vi "rqcAlice Key Distribution (Low Level Example).vi"() -> ()   [LabVIEW 2018]
uses:
  Custom Controls/rqcAlice States.ctl
  FPGA/Alice/Custom Controls/Phase Modulator/rqcAlice Mod.Config.ctl
  Shared/Shared FPGA Lib/Shared Logic/Custom Controls/rqc Random Generator.parameters.ctl
  Shared/Shared FPGA Lib/Shared Logic/Custom Controls/rqc Random Generator.value type.ctl
  FPGA/Alice/Custom Controls/Main State Machine/rqcAlice DAC Clock Positions.ctl
  Shared/Shared Host Lib/rqc ServiceNET/Custom Controls/rqc ServiceNET command.ctl
  Shared/Shared Host Lib/rqc ServiceNET/Alice/Custom Controls/rqcAlice ServiceNET control.ctl
  <vilib>/FPGAPlugInAG/PCIe-7820R/niLvFpga_Open_PCIe-7820R.vi
  <vilib>/rvi/interface/common/dynamic/niFpgaDynamicAddResources.vi
  <vilib>/FPGAPlugInAG/Dynamic/niLvFpga_Close_Dynamic.vi
  <vilib>/rvi/interface/nirviOpenFPGA/nirviOpenFPGA.xnode
  FPGA Bitfiles/rqcAlice FPGA (7820R) v 3.2.0.lvbitx
  <vilib>/rvi/interface/nirviCloseFPGA/nirviCloseFPGA.xnode
panel:
  in  "Sessions to Key File":u32
  in  "Write to File QBER threshold":dbl=5.0 format="%#_g %"
  in  "Attenuation, dB":dbl max=40.0
  out "IP Address":string="192.168.0.209"
  in  "DL SD":u32=24674
  in  "Coax/SD":bool
  out "QBER Graph":dbl[](graph)
  in  "pm.off":u8=2
  in  "pm.on":u8=9
  in  "PM\nRandom\nOn/Off":bool=TRUE
  in  "Pi Voltage":u16=160
  out "Real pulse count:":i32=1000000
  out "Total pulses expected:":u32=1000000
  out "QBER, %":dbl=1.8333333333333333
  out "Bob's Key:":string="000001111000001000111001111011010101010110101010000001111011010111010100010111101101000100111011011011100011101010101111010000010101011111010011110111101011110110111011001100100110010000110101011100111010010011100011011100000100000100011001010111010011011011011111001000001100001100101000101111000011101010000011011101000010000001100110010111011010110010111010010100010111010010111010010010101000110110111000000101101000010001111111011110101110001110011010101111011010011001011111000111111101001100010111110011011101111001111000111010111111101001001100001111010010001111001011101101001000000101001010"
  out "Alice's Key:":string="000001111000001000111000111011010101010110101010000001111011010111010100010111101001000110111011011011100011101010101111010010010101011111010011110111101011111110111011001100100110010000110101011100111010010011100011011100000100000100011001110111010011011011011101001000001100001100101000101111000011100010000011011101000010000001100010110111011010110010111010010100010111010010111010010010101000110110111000000101101000010001111111011110101110001110011010101111011010011001011111000111111101001100010111110011011101111001111000111010111111101001001100001111010010001111001011111101001000000101001010"
  in  "Pulses in Train":u32=1000
  in  "Train Number":i32=1000
  in  "DL Coax":u32=24704
  out "error out":errorcluster
  in  "Stop":bool
  out "connected?":bool
  in  "Port":u16=5020
  out "Current State":T1=enum."App.Stop"
  # "ALICE"
  # "LAN settings:"
  # "Data exchange details:"
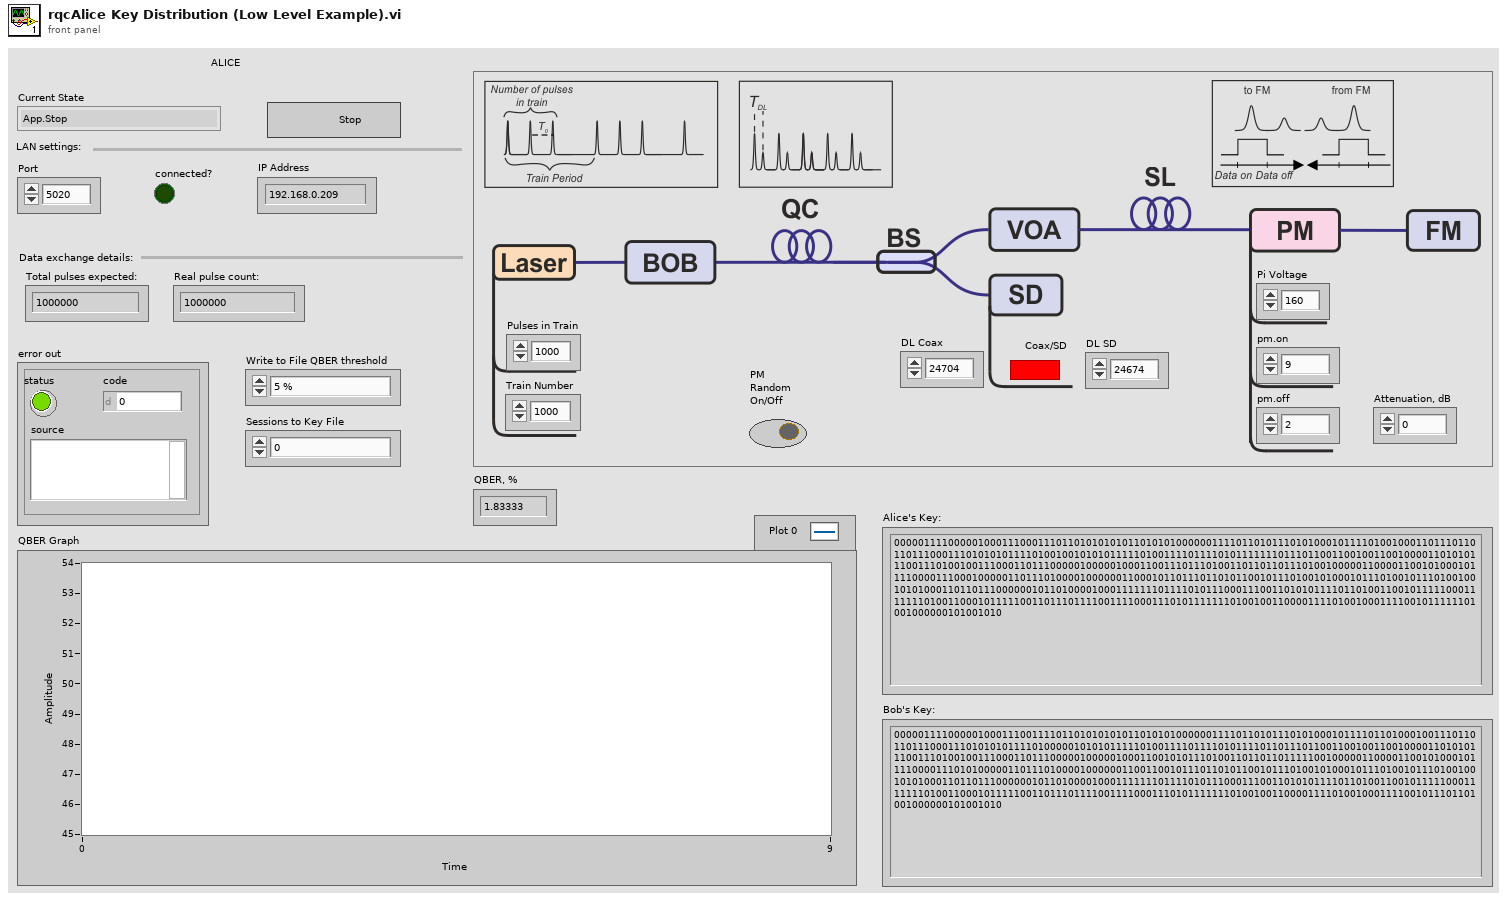
[diagram p1: front panel]
types:
  T1 = typedef "rqcAlice States.ctl" = enum16{"HW.configure", "HW.meas", "NET.create", "NET.connect", "NET.readCommand", "NET.sendCommand", "NET.readData", "NET.close", "Meas.Start", "Meas.NextStep", "Meas.restart", "Meas.Done", "App.HandleEvent", "App.HandleError", "App.Stop"}
  T2 = typedef "rqcAlice DAC Clock Positions.ctl" = u8[]
  T3 = typedef "rqc Random Generator.parameters.ctl" = cluster{"value type":T4, "constant":u16, "num of levels":u16, "levels values":u16[]}
  T4 = typedef "rqc Random Generator.value type.ctl" = enum16{"random value", "constant"}
  T5 = typedef "rqcAlice Mod.Config.ctl" = cluster{"mod.on":u8, "mod.off":u8}
  T6 = typedef "rqc ServiceNET command.ctl" = enum8{"NONE", "READY", "START", "PING", "SEND KEY", "WRITE KEY", "WRITE AND SAVE KEY"}
  T7 = typedef "rqcAlice ServiceNET control.ctl" = cluster{"connection ID":refnum<k5>, "port":u16, "connected?":bool}
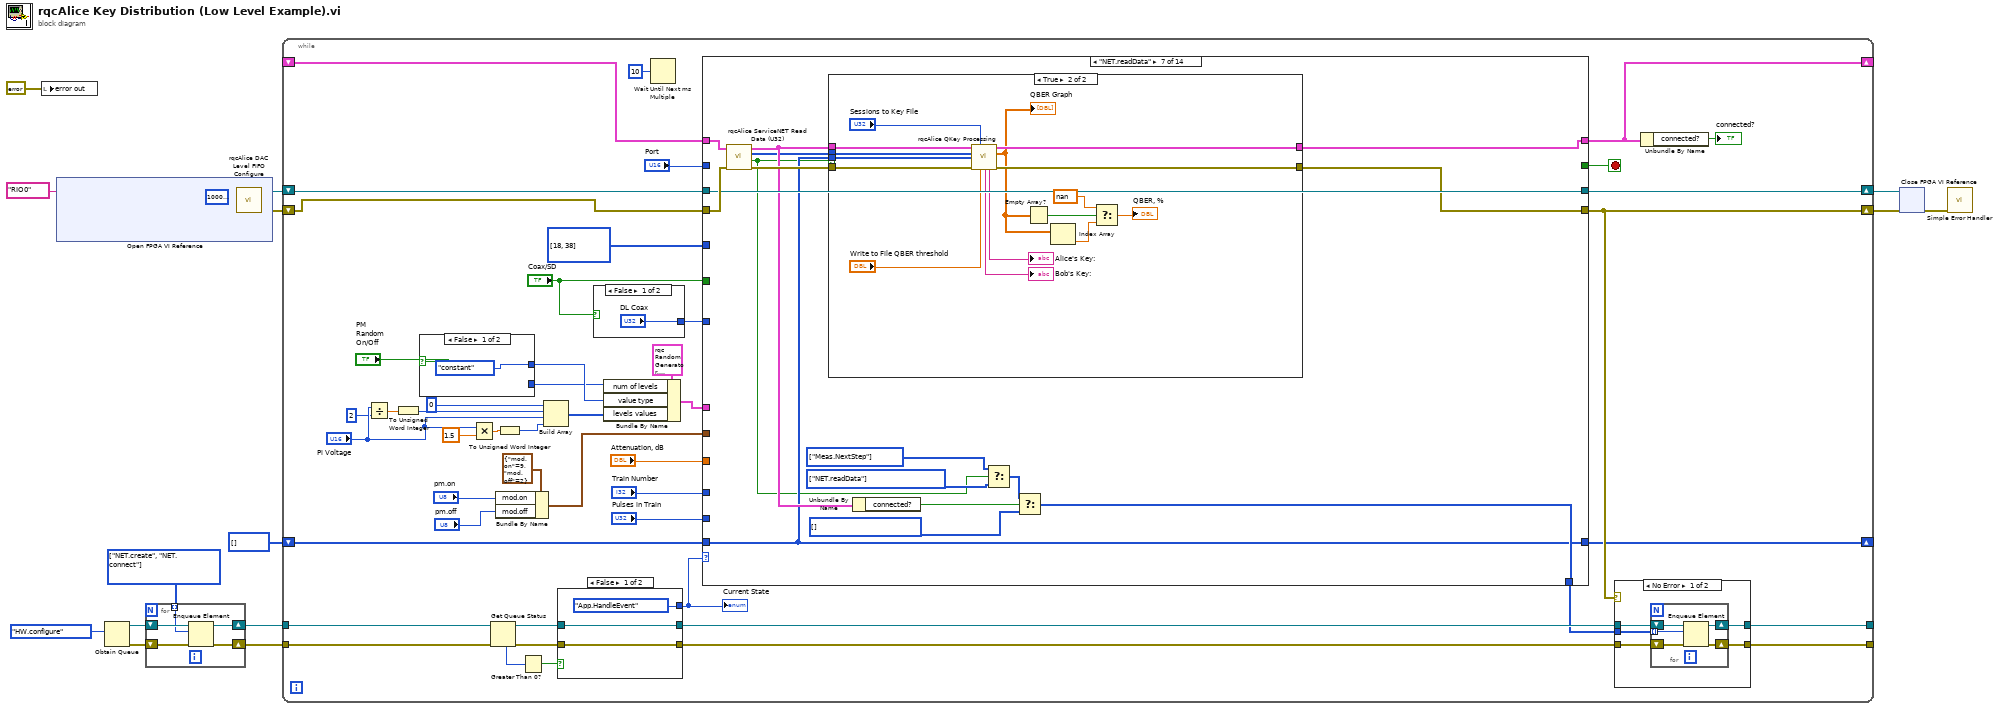
[diagram p0: block diagram]
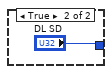
[diagram p2: hidden frame]
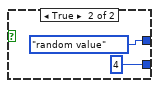
[diagram p3: hidden frame]
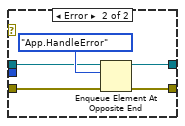
[diagram p4: hidden frame]
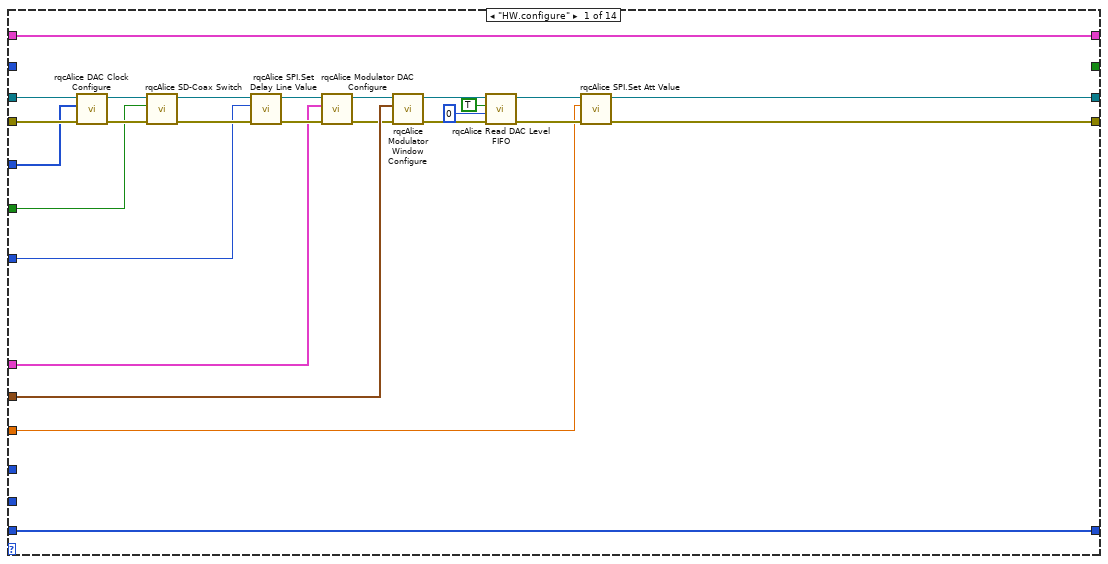
[diagram p5: hidden frame]
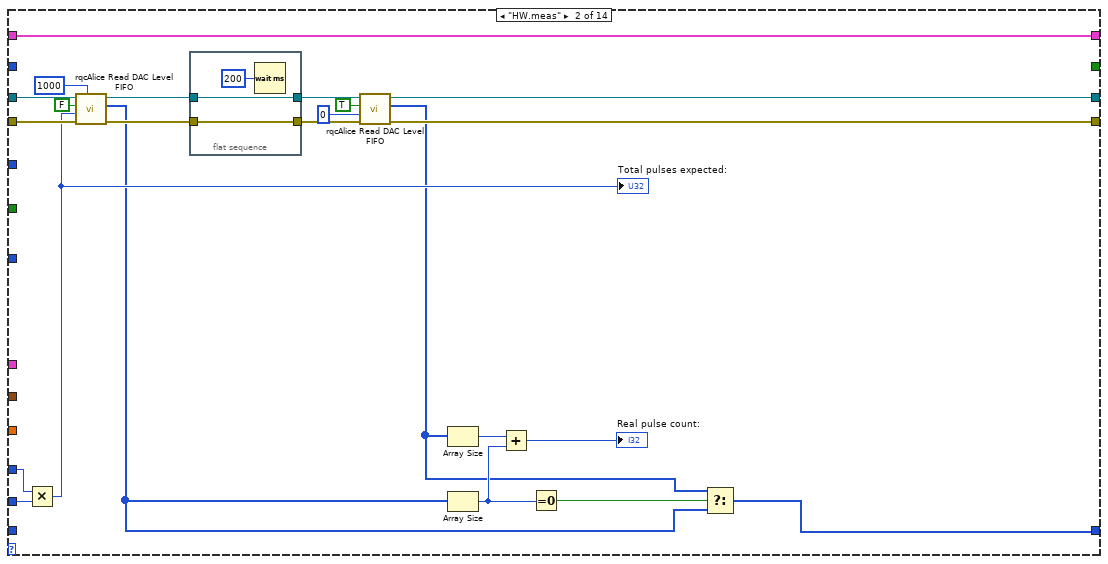
[diagram p6: hidden frame]
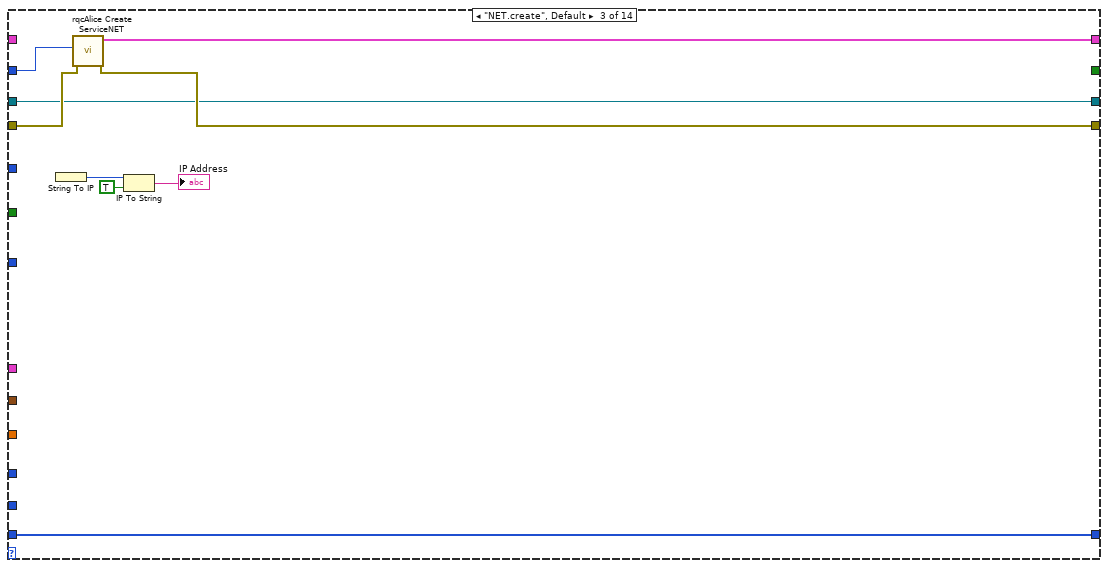
[diagram p7: hidden frame]
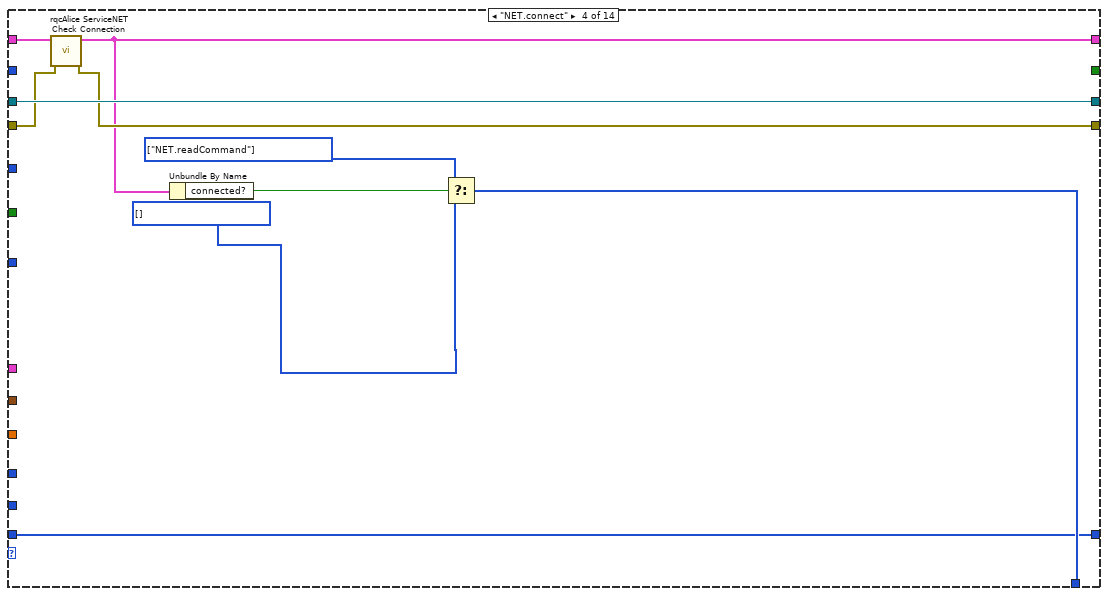
[diagram p8: hidden frame]
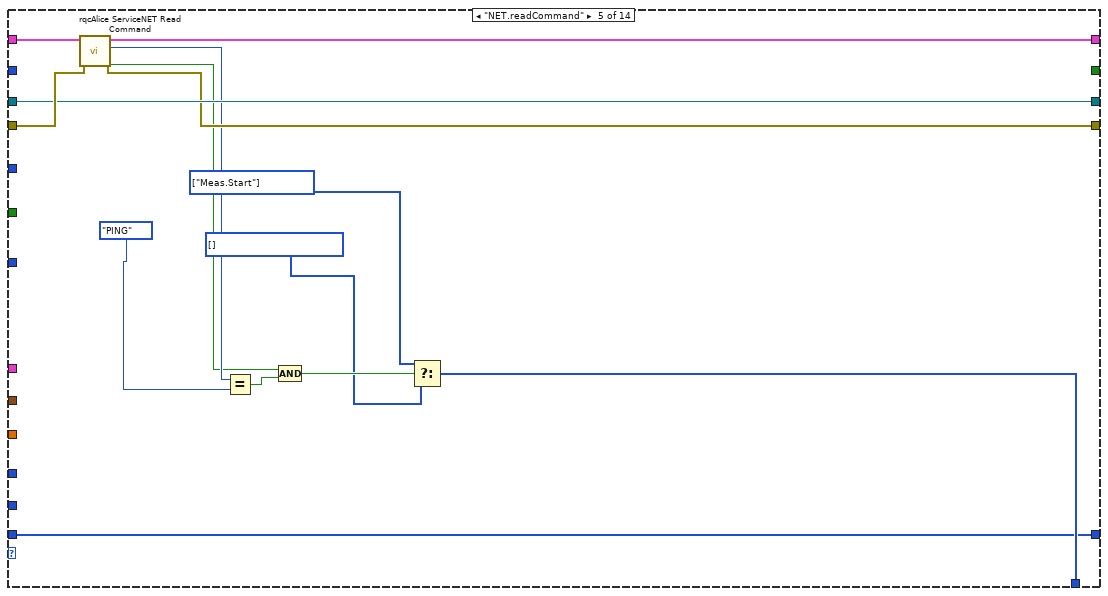
[diagram p9: hidden frame]
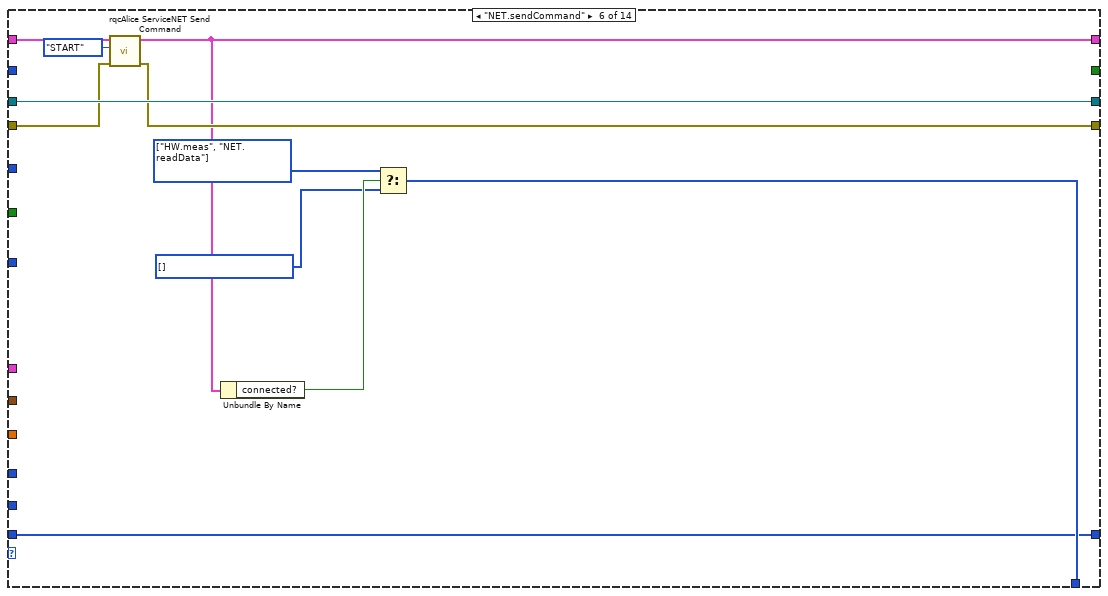
[diagram p10: hidden frame]
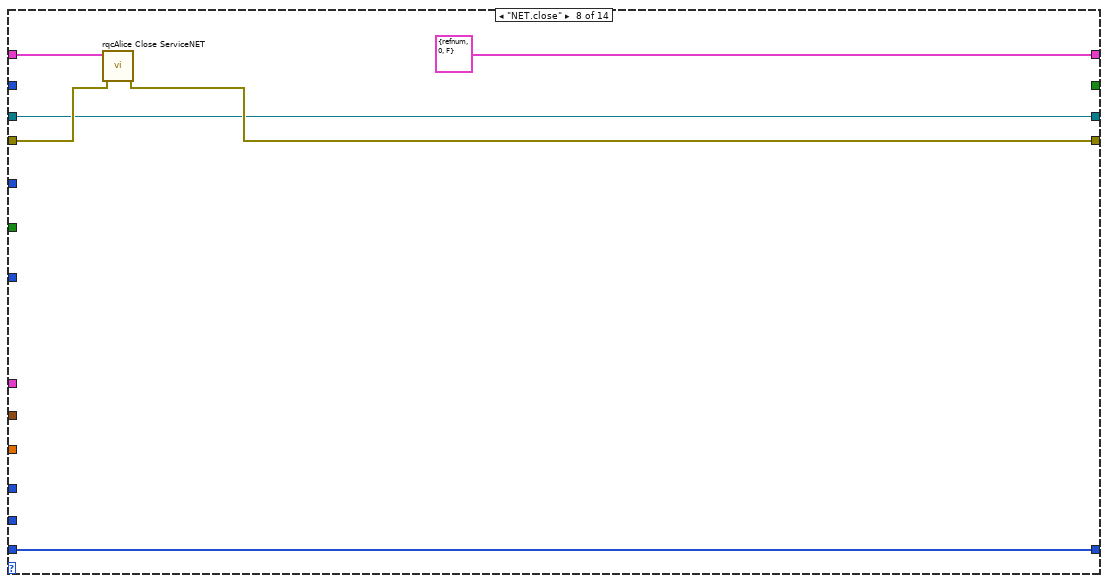
[diagram p12: hidden frame]
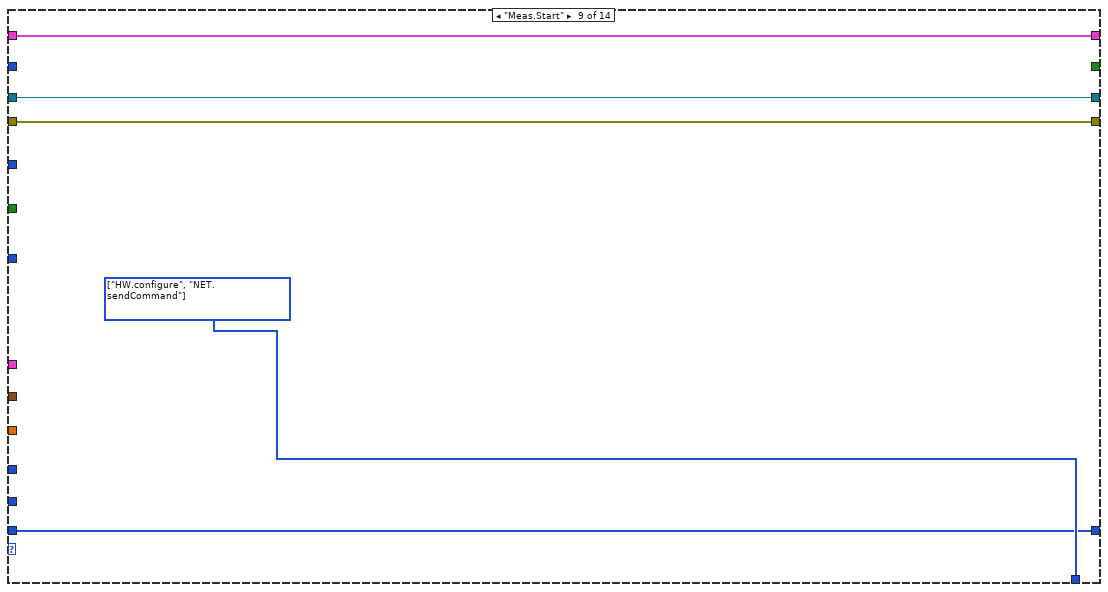
[diagram p13: hidden frame]
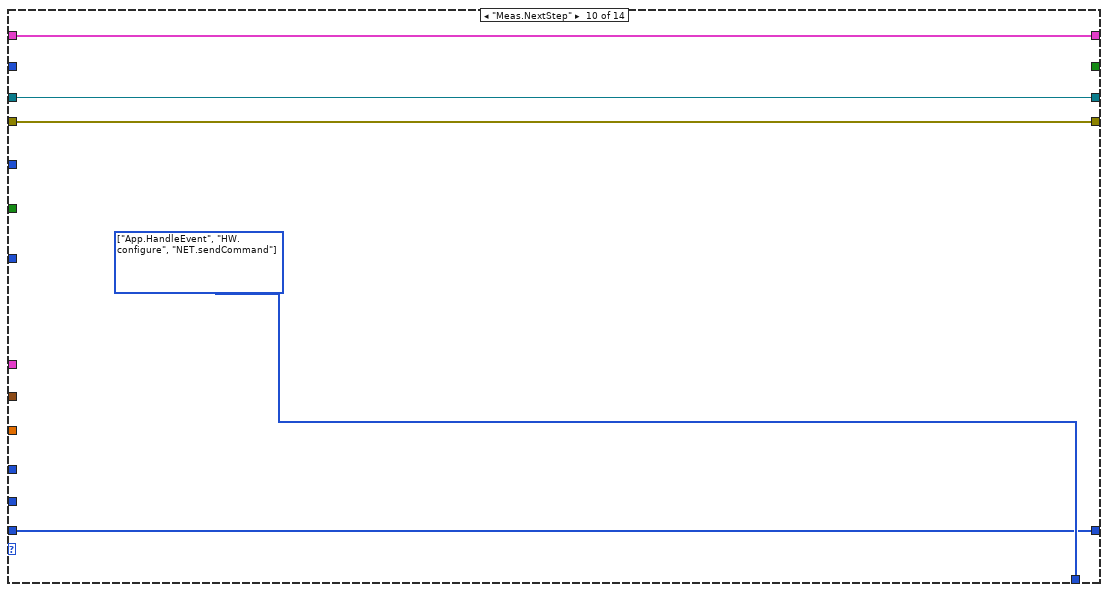
[diagram p14: hidden frame]
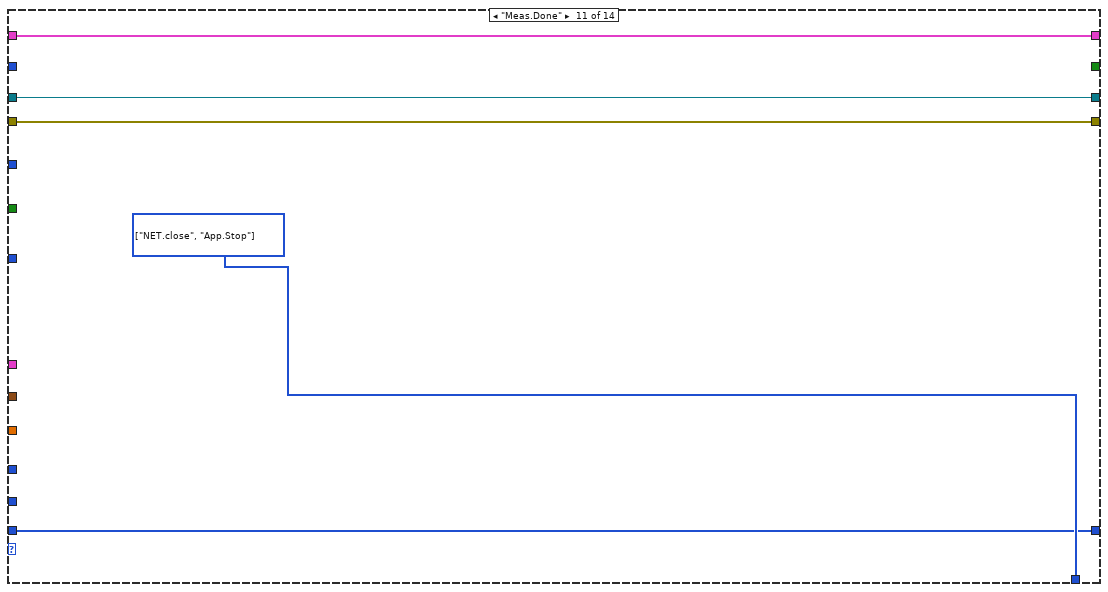
[diagram p15: hidden frame]
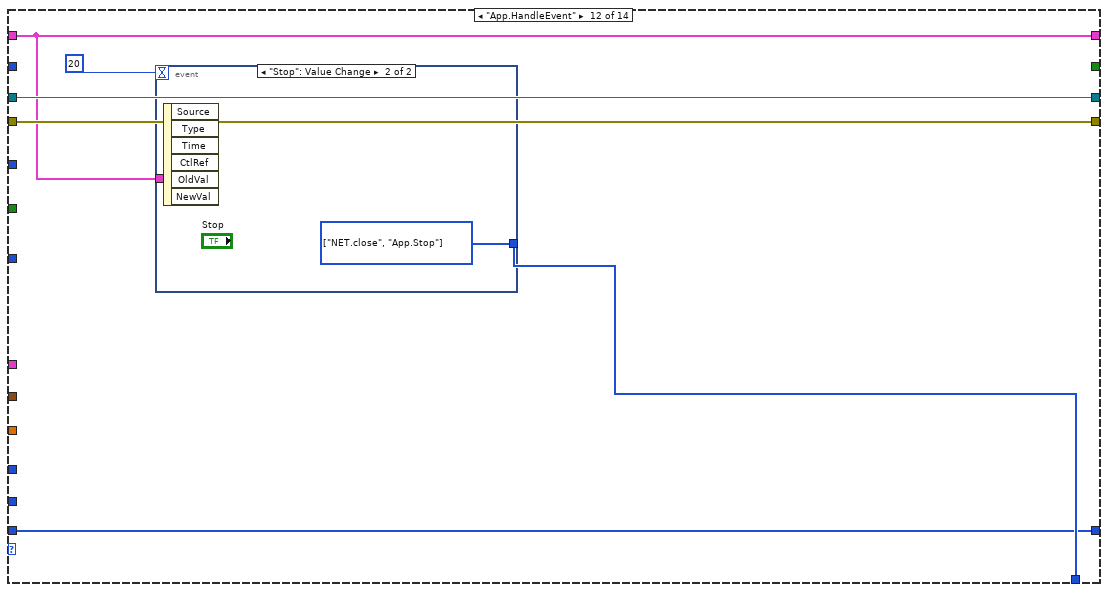
[diagram p16: hidden frame]
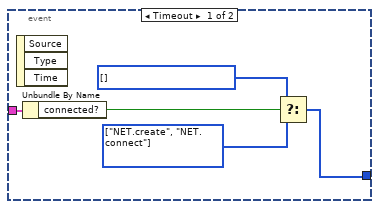
[diagram p17: hidden frame]
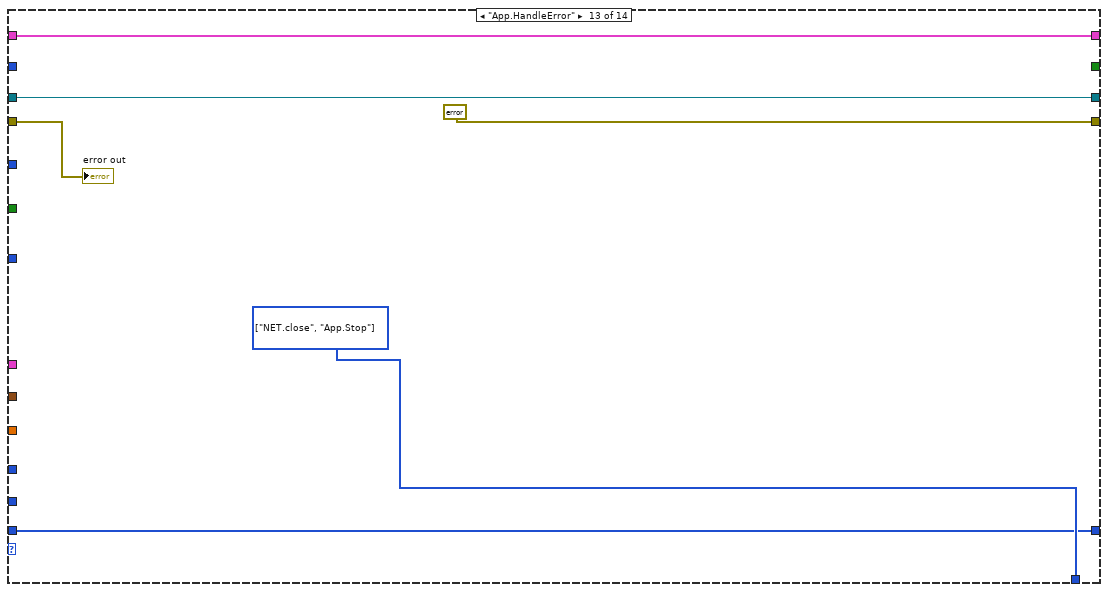
[diagram p18: hidden frame]
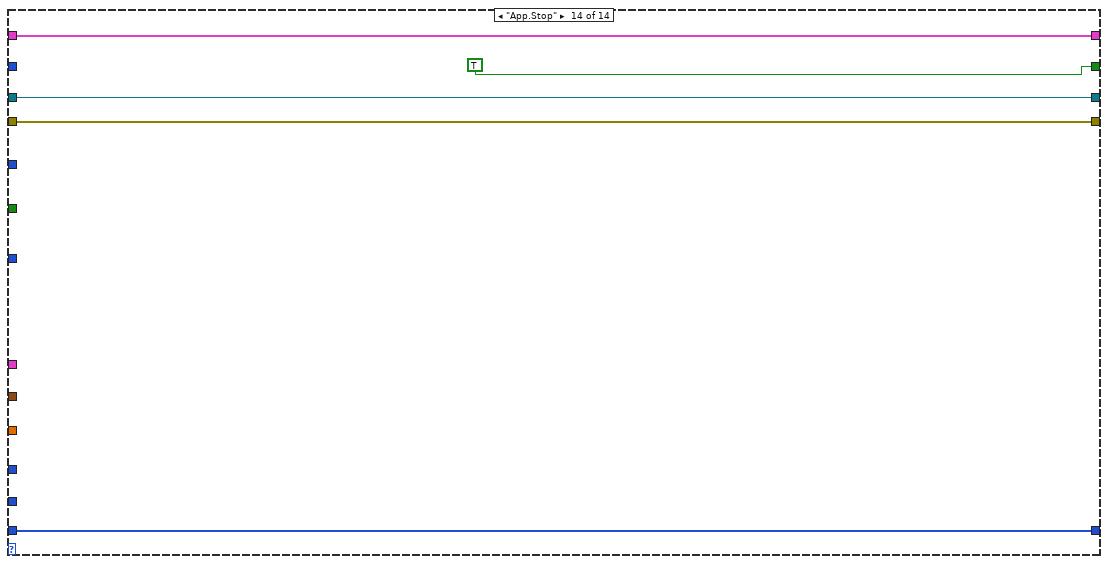
[diagram p19: hidden frame]
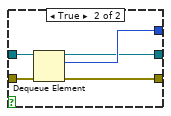
[diagram p20: hidden frame]
diagram:
  w11 = T1[] [enum."NET.create", enum."NET.connect"] items=["HW.configure", "HW.meas", "NET.create", "NET.connect", "NET.readCommand", "NET.sendCommand", "NET.readData", "NET.close", "Meas.Start", "Meas.NextStep", "Meas.restart", "Meas.Done", "App.HandleEvent", "App.HandleError", "App.Stop"]
  n1 = local write "error out"(errorcluster {"status"=FALSE, "code"=0, "source"=""} ("error out")) -> ()
  n2 = xnode "Open FPGA VI Reference"("resource name"=tag "RIO0") -> ("FPGA VI Reference Out"=w6:refnum<k20>, "error out"=w4:errorcluster)  [unwired: 1 in]
  n3 = Obtain Queue(element data type=rqcAlice_States."HW.configure" ("rqcAlice States")) -> (queue out=w13:refnum<queue>, error out=w12:errorcluster)  [unwired: 4 in, 1 out]
  n4 = for {
    shift-right: [w20] -> w10
    shift-left: w13 -> [w22]
    shift-right: [w19] -> w9
    shift-left: w12 -> [w21]
    tunnel: w11 -> [w18] mode=indexing
    n5 = Enqueue Element(queue=w22, element=w18, error in (no error)=w21) -> (queue out=w20:refnum<queue>, error out=w19:errorcluster)  [unwired: 1 in, 1 out]
  }
  n6 = call "rqcAlice DAC Level FIFO Configure.vi"("error in"=w4, "DAC Level FIFO Depth"=u32 10000000, "Alice FPGA Reference In"=w6) -> ("error out"=w3:errorcluster, "Alice FPGA Reference Out"=w5:refnum<k20>)  [unwired: 7 in]
  n7 = while {
    tunnel: w10 -> [w69]
    shift-right: [w70] -> w16
    shift-left: w5 -> [w32]
    shift-right: [w62] -> w15
    shift-left: w3 -> [w31]
    tunnel: w9 -> [w68]
    tunnel: [w59] -> _
    tunnel: [w58] -> _
    shift-right: [w54] -> _
    shift-left: _ -> [w56]
    shift-right: [w48] -> _
    shift-left: u8[] [] ("Data") -> [w47]
    stop <- w52 stop-if-true
    n8 = Divide(x="Pi Voltage", y=2) -> (x/y=w39:dbl)
    n9 = To Unsigned Word Integer(number=w39) -> (unsigned 16bit integer=w44:u16)
    n10 = case shown="False" "PM\nRandom\nOn/Off" {
      tunnel: [rqc_Random_Generator.value_type."constant" ("pm.value type") rqc_Random_Generator.value_type."random value" ("pm.value type")] -> w37
      tunnel: [_ u16 4 ("num of levels")] -> w23
      frame False {
      }
      frame True {
      }
    }
    n11 = Multiply(x="Pi Voltage", y=1.5) -> (x*y=w41:dbl)
    n12 = Get Queue Status(queue=w69, error in (no error)=w68) -> (queue out=w65:refnum<queue>, error out=w64:errorcluster, # elements in queue=w67:i32)  [unwired: 1 in, 5 out]
    n13 = Bundle By Name(cluster=T5 {"mod.on"=9, "mod.off"=2} ("Modulator config"), "mod.on"="pm.on", "mod.off"="pm.off") -> (w26:T5)
    n14 = To Unsigned Word Integer(number=w41) -> (unsigned 16bit integer=w46:u16)
    n15 = Greater Than 0?(x=w67) -> (x > 0?=w66:bool)
    n16 = Build Array(u16 0 ("element"), w44, "Pi Voltage", w46) -> (w36:u16[])
    n17 = case shown="False" w66 {
      tunnel: w65 -> [w265 w271]
      tunnel: w64 -> [w264 w270]
      tunnel: [rqcAlice_States."App.HandleEvent" ("rqcAlice States") w269] -> w63
      tunnel: [w265 w268] -> w61
      tunnel: [w264 w267] -> w60
      frame False {
      }
      frame True {
        n18 = Dequeue Element(queue=w271, error in (no error)=w270) -> (queue out=w268:refnum<queue>, element=w269:T1, error out=w267:errorcluster)  [unwired: 1 in, 1 out]
      }
    }
    "Current State" <- w63
    n19 = case shown="False" "Coax/SD" {
      tunnel: ["DL Coax" "DL SD"] -> w33
      frame False {
      }
      frame True {
      }
    }
    n20 = Bundle By Name(cluster=T3 {"value type"=enum."random value", "constant"=150, "num of levels"=4, "levels values"=[0, 75, 150, 225]} ("RndGen.parameters"), "num of levels"=w23, "value type"=w37, "levels values"=w36) -> (w28:T3)
    n21 = Wait Until Next ms Multiple(millisecond multiple=u32 10) -> ()  [unwired: 1 out]
    n22 = case shown="\"NET.readData\"" w63 {
      tunnel: w32 -> [w116 w139 w148 w161 w172 w186 w200 w221 w229 w234 w239 w246 w257 w262]
      tunnel: w31 -> [w115 w138 w150 w159 w174 w184 w201 w224 w228 w233 w238 w245 w256 w261]
      tunnel: w26 -> [w114 _ _ _ _ _ _ _ _ _ _ _ _ _]
      tunnel: [w99 w131 w148 w161 w172 w186 w200 w221 w229 w234 w239 w246 w257 w262] -> w70
      tunnel: [w97 w130 w149 w158 w171 w183 w192 w223 w228 w233 w238 w245 errorcluster {"status"=FALSE, "code"=0, "source"=""} ("error out") w261] -> w62
      tunnel: [_ _ _ w154 w163 w177 w194 _ w227 w232 w237 w242 w254 _] -> w57
      tunnel: [w113 w134 w151 w157 w173 w181 w191 T7 {"connection ID"=refnum, "port"=0, "connected?"=FALSE} ("rqcAlice ServiceNET out") w230 w235 w240 w243 w258 w260] -> w54
      tunnel: w56 -> [w113 w134 _ w160 w175 w185 w202 w225 w230 w235 w240 w243 w258 w260]
      tunnel: "Port" -> [_ _ w147 _ _ _ _ _ _ _ _ _ _ _]
      tunnel: [_ _ _ _ _ _ _ _ _ _ _ _ _ TRUE] -> w52
      tunnel: w33 -> [w101 _ _ _ _ _ _ _ _ _ _ _ _ _]
      tunnel: "Train Number" -> [_ w137 _ _ _ _ _ _ _ _ _ _ _ _]
      tunnel: "Pulses in Train" -> [_ w136 _ _ _ _ _ _ _ _ _ _ _ _]
      tunnel: [w112 w121 w146 w152 w162 w176 w188 w220 w226 w231 w236 w241 w253 w259] -> w48
      tunnel: w47 -> [w112 _ w146 w152 w162 w176 w188 w220 w226 w231 w236 w241 w253 w259]
      tunnel: T2 [18, 38] ("DAC Clock params") -> [w109 _ _ _ _ _ _ _ _ _ _ _ _ _]
      tunnel: w28 -> [w93 _ _ _ _ _ _ _ _ _ _ _ _ _]
      tunnel: "Coax/SD" -> [w104 _ _ _ _ _ _ _ _ _ _ _ _ _]
      tunnel: "Attenuation, dB" -> [w96 _ _ _ _ _ _ _ _ _ _ _ _ _]
      frame "HW.configure" {
        n23 = call "rqcAlice DAC Clock Configure.vi"("error in"=w115, "DAC Clock params"=w109, "Alice FPGA Reference In"=w116) -> ("error out"=w105:errorcluster, "Alice FPGA Reference Out"=w106:refnum<k20>)  [unwired: 7 in]
        n24 = call "rqcAlice SD-Coax Switch.vi"("error in"=w105, "SD/Coax Select"=w104, "Alice FPGA Reference In"=w106) -> ("error out"=w102:errorcluster, "Alice FPGA Reference Out"=w103:refnum<k20>)  [unwired: 7 in]
        n25 = call "rqcAlice SPI.Set Delay Line Value.vi"("error in"=w102, "Delay Line Value"=w101, "Alice FPGA Reference In"=w103) -> ("error out"=w94:errorcluster, "Alice FPGA Reference Out"=w95:refnum<k20>)  [unwired: 7 in]
        n26 = call "rqcAlice Modulator DAC Configure.vi"("error in"=w94, "RndGen.parameters"=w93, "Alice FPGA Reference In"=w95) -> ("error out"=w92:errorcluster, "Alice FPGA Reference Out"=w91:refnum<k20>)  [unwired: 7 in]
        n27 = call "rqcAlice Modulator Window Configure.vi"("error in"=w92, "Modulator config"=w114, "Alice FPGA Reference In"=w91) -> ("error out"=w108:errorcluster, "Alice FPGA Reference Out"=w107:refnum<k20>)  [unwired: 7 in]
        n28 = call "rqcAlice Read DAC Level FIFO.vi"("error in"=w108, "number of elements"=u32 0, "read all available"=TRUE, "Alice FPGA Reference In"=w107) -> ("error out"=w98:errorcluster, "Alice FPGA Reference Out"=w100:refnum<k20>)  [unwired: 4 in, 2 out]
        n29 = call "rqcAlice SPI.Set Att Value.vi"("error in"=w98, "Attenuation, dB"=w96, "Alice FPGA Reference In"=w100) -> ("error out"=w97:errorcluster, "Alice FPGA Reference Out"=w99:refnum<k20>)  [unwired: 7 in]
      }
      frame "HW.meas" {
        n30 = Multiply(x=w137, y=w136) -> (x*y=w133:u32)
        "Total pulses expected:" <- w133
        n31 = call "rqcAlice Read DAC Level FIFO.vi"("timeout (ms)"=1000, "error in"=w138, "number of elements"=w133, "read all available"=FALSE, "Alice FPGA Reference In"=w139) -> ("error out"=w127:errorcluster, "Data"=w125:u8[], "Alice FPGA Reference Out"=w126:refnum<k20>)  [unwired: 3 in, 1 out]
        n32 = flat-sequence {
          tunnel: [w142] -> w118
          tunnel: w127 -> [w142]
          tunnel: [w141] -> w117
          tunnel: w126 -> [w141]
          frame #0 {
            n33 = Wait (ms)(milliseconds to wait=u32 200) -> ()  [unwired: 1 out]
          }
        }
        n34 = call "rqcAlice Read DAC Level FIFO.vi"("error in"=w118, "number of elements"=u32 0, "read all available"=TRUE, "Alice FPGA Reference In"=w117) -> ("error out"=w130:errorcluster, "Data"=w122:u8[], "Alice FPGA Reference Out"=w131:refnum<k20>)  [unwired: 4 in, 1 out]
        n35 = Array Size(array=w122) -> (size(s)=w128:i32)
        n36 = Array Size(array=w125) -> (size(s)=w124:i32)
        n37 = Add(x=w128, y=w124) -> (x+y=→"Real pulse count:":i32)
        n38 = Equal To 0?(x=w124) -> (x = 0?=w123:bool)
        n39 = Select(t=w122, s=w123, f=w125) -> (s? t:f=w121:u8[])
      }
      frame "NET.create", Default {
        n40 = String To IP() -> (0:w144:u32)  [unwired: 1 in]
        n41 = call "rqcAlice Create ServiceNET.vi"("error in"=w150, "port"=w147) -> ("error out"=w149:errorcluster, "rqcAlice ServiceNET control"=w151:T7)  [unwired: 8 in]
        n42 = IP To String(1:TRUE ("dot notation? (F)"), 2:w144) -> (0:→"IP Address":string)
      }
      frame "NET.connect" {
        w153 = T1[] [] items=["HW.configure", "HW.meas", "NET.create", "NET.connect", "NET.readCommand", "NET.sendCommand", "NET.readData", "NET.close", "Meas.Start", "Meas.NextStep", "Meas.restart", "Meas.Done", "App.HandleEvent", "App.HandleError", "App.Stop"] ("f")
        w155 = T1[] [enum."NET.readCommand"] items=["HW.configure", "HW.meas", "NET.create", "NET.connect", "NET.readCommand", "NET.sendCommand", "NET.readData", "NET.close", "Meas.Start", "Meas.NextStep", "Meas.restart", "Meas.Done", "App.HandleEvent", "App.HandleError", "App.Stop"]
        n43 = call "rqcAlice ServiceNET Check Connection.vi"("error in"=w159, "rqcAlice ServiceNET in"=w160) -> ("error out"=w158:errorcluster, "rqcAlice ServiceNET out"=w157:T7)  [unwired: 8 in]
        n44 = Unbundle By Name(w157) -> ("connected?"=w156:bool)
        n45 = Select(t=w155, s=w156, f=w153) -> (s? t:f=w154:T1[])
      }
      frame "NET.readCommand" {
        w164 = T1[] [] items=["HW.configure", "HW.meas", "NET.create", "NET.connect", "NET.readCommand", "NET.sendCommand", "NET.readData", "NET.close", "Meas.Start", "Meas.NextStep", "Meas.restart", "Meas.Done", "App.HandleEvent", "App.HandleError", "App.Stop"] ("f")
        w165 = T1[] [enum."Meas.Start"] items=["HW.configure", "HW.meas", "NET.create", "NET.connect", "NET.readCommand", "NET.sendCommand", "NET.readData", "NET.close", "Meas.Start", "Meas.NextStep", "Meas.restart", "Meas.Done", "App.HandleEvent", "App.HandleError", "App.Stop"] ("f")
        n46 = call "rqcAlice ServiceNET Read Command.vi"("error in"=w174, "rqcAlice ServiceNET in"=w175) -> ("error out"=w171:errorcluster, "cmd valid"=w167:bool, "command"=w169:T6, "rqcAlice ServiceNET out"=w173:T7)  [unwired: 6 in]
        n47 = Equal?(x=w169, y=rqc_ServiceNET_command."PING" ("command")) -> (x = y?=w168:bool)
        n48 = Compound Arithmetic op=AND(w167, w168) -> (w166:bool)
        n49 = Select(t=w165, s=w166, f=w164) -> (s? t:f=w163:T1[])
      }
      frame "NET.sendCommand" {
        w178 = T1[] [] items=["HW.configure", "HW.meas", "NET.create", "NET.connect", "NET.readCommand", "NET.sendCommand", "NET.readData", "NET.close", "Meas.Start", "Meas.NextStep", "Meas.restart", "Meas.Done", "App.HandleEvent", "App.HandleError", "App.Stop"] ("f")
        w179 = T1[] [enum."HW.meas", enum."NET.readData"] items=["HW.configure", "HW.meas", "NET.create", "NET.connect", "NET.readCommand", "NET.sendCommand", "NET.readData", "NET.close", "Meas.Start", "Meas.NextStep", "Meas.restart", "Meas.Done", "App.HandleEvent", "App.HandleError", "App.Stop"] ("f")
        n50 = call "rqcAlice ServiceNET Send Command.vi"("error in"=w184, "command"=rqc_ServiceNET_command."START", "rqcAlice ServiceNET in"=w185) -> ("error out"=w183:errorcluster, "rqcAlice ServiceNET out"=w181:T7)  [unwired: 7 in]
        n51 = Unbundle By Name(w181) -> ("connected?"=w180:bool)
        n52 = Select(t=w179, s=w180, f=w178) -> (s? t:f=w177:T1[])
      }
      frame "NET.readData" {
        w195 = T1[] [] items=["HW.configure", "HW.meas", "NET.create", "NET.connect", "NET.readCommand", "NET.sendCommand", "NET.readData", "NET.close", "Meas.Start", "Meas.NextStep", "Meas.restart", "Meas.Done", "App.HandleEvent", "App.HandleError", "App.Stop"] ("f")
        w199 = T1[] [enum."Meas.NextStep"] items=["HW.configure", "HW.meas", "NET.create", "NET.connect", "NET.readCommand", "NET.sendCommand", "NET.readData", "NET.close", "Meas.Start", "Meas.NextStep", "Meas.restart", "Meas.Done", "App.HandleEvent", "App.HandleError", "App.Stop"] ("t")
        w198 = T1[] [enum."NET.readData"] items=["HW.configure", "HW.meas", "NET.create", "NET.connect", "NET.readCommand", "NET.sendCommand", "NET.readData", "NET.close", "Meas.Start", "Meas.NextStep", "Meas.restart", "Meas.Done", "App.HandleEvent", "App.HandleError", "App.Stop"] ("f")
        n53 = call "rqcAlice ServiceNET Read Data (U32).vi"("error in"=w201, "rqcAlice ServiceNET in"=w202) -> ("error out"=w193:errorcluster, "data valid"=w187:bool, "data"=w189:u32[], "rqcAlice ServiceNET out"=w190:T7)  [unwired: 6 in]
        n54 = case shown="True" w187 {
          tunnel: w193 -> [w203 w219]
          tunnel: [w203 w218] -> w192
          tunnel: [w204 w217] -> w191
          tunnel: w190 -> [w204 w216]
          tunnel: w189 -> [_ w215]
          tunnel: w188 -> [_ w214]
          frame False {
          }
          frame True {
            n55 = call "rqcAlice QKey Processing.vi"("rqcAlice ServiceNET in"=w216, "Sessions to Key File"="Sessions to Key File", "Bob's data"=w215, "Alice's Raw data"=w214, "error in (no error)"=w219, "Write to File QBER threshold"="Write to File QBER threshold") -> ("rqcAlice ServiceNET out"=w217:T7, "QBER, %"=w209:dbl[], "Bob's Key:"=→"Bob's Key:":string, "Alice's Key:"=→"Alice's Key:":string, "error out"=w218:errorcluster)  [unwired: 5 in]
            "QBER Graph" <- w209
            n56 = Empty Array?(array=w209) -> (empty?=w208:bool)
            n57 = Index Array(array=w209) -> (element=w207:dbl)  [unwired: 1 in]
            n58 = Select(t=nan, s=w208, f=w207) -> (s? t:f=→"QBER, %":dbl)
          }
        }
        n59 = Unbundle By Name(w190) -> ("connected?"=w197:bool)
        n60 = Select(t=w199, s=w187, f=w198) -> (s? t:f=w196:T1[])
        n61 = Select(t=w196, s=w197, f=w195) -> (s? t:f=w194:T1[])
      }
      frame "NET.close" {
        n62 = call "rqcAlice Close ServiceNET.vi"("error in"=w224, "rqcAlice ServiceNET in"=w225) -> ("error out"=w223:errorcluster)  [unwired: 9 in]
      }
      frame "Meas.Start" {
        w227 = T1[] [enum."HW.configure", enum."NET.sendCommand"] items=["HW.configure", "HW.meas", "NET.create", "NET.connect", "NET.readCommand", "NET.sendCommand", "NET.readData", "NET.close", "Meas.Start", "Meas.NextStep", "Meas.restart", "Meas.Done", "App.HandleEvent", "App.HandleError", "App.Stop"] ("f")
      }
      frame "Meas.NextStep" {
        w232 = T1[] [enum."App.HandleEvent", enum."HW.configure", enum."NET.sendCommand"] items=["HW.configure", "HW.meas", "NET.create", "NET.connect", "NET.readCommand", "NET.sendCommand", "NET.readData", "NET.close", "Meas.Start", "Meas.NextStep", "Meas.restart", "Meas.Done", "App.HandleEvent", "App.HandleError", "App.Stop"] ("f")
      }
      frame "Meas.Done" {
        w237 = T1[] [enum."NET.close", enum."App.Stop"] items=["HW.configure", "HW.meas", "NET.create", "NET.connect", "NET.readCommand", "NET.sendCommand", "NET.readData", "NET.close", "Meas.Start", "Meas.NextStep", "Meas.restart", "Meas.Done", "App.HandleEvent", "App.HandleError", "App.Stop"] ("f")
      }
      frame "App.HandleEvent" {
        n63 = event shown="[1] \"Stop\": Value Change" {
          selector: _ -> [_ _]
          dyn-events: _ -> [_ _]
          timeout: 20 -> [_ _]
          tunnel: w243 -> [w251 _]
          tunnel: [w247 w252] -> w242
          event Timeout {
            w248 = T1[] [enum."NET.create", enum."NET.connect"] items=["HW.configure", "HW.meas", "NET.create", "NET.connect", "NET.readCommand", "NET.sendCommand", "NET.readData", "NET.close", "Meas.Start", "Meas.NextStep", "Meas.restart", "Meas.Done", "App.HandleEvent", "App.HandleError", "App.Stop"]
            w249 = T1[] [] items=["HW.configure", "HW.meas", "NET.create", "NET.connect", "NET.readCommand", "NET.sendCommand", "NET.readData", "NET.close", "Meas.Start", "Meas.NextStep", "Meas.restart", "Meas.Done", "App.HandleEvent", "App.HandleError", "App.Stop"]
            n64 = event-data() -> ()  [unwired: 1 in, 3 out]
            n65 = Unbundle By Name(w251) -> ("connected?"=w250:bool)
            n66 = Select(t=w249, s=w250, f=w248) -> (s? t:f=w247:T1[])
          }
          event "Stop": Value Change {
            w252 = T1[] [enum."NET.close", enum."App.Stop"] items=["HW.configure", "HW.meas", "NET.create", "NET.connect", "NET.readCommand", "NET.sendCommand", "NET.readData", "NET.close", "Meas.Start", "Meas.NextStep", "Meas.restart", "Meas.Done", "App.HandleEvent", "App.HandleError", "App.Stop"]
            n67 = event-data() -> ()  [unwired: 1 in, 6 out]
          }
        }
      }
      frame "App.HandleError" {
        w254 = T1[] [enum."NET.close", enum."App.Stop"] items=["HW.configure", "HW.meas", "NET.create", "NET.connect", "NET.readCommand", "NET.sendCommand", "NET.readData", "NET.close", "Meas.Start", "Meas.NextStep", "Meas.restart", "Meas.Done", "App.HandleEvent", "App.HandleError", "App.Stop"] ("f")
        "error out" <- w256
      }
      frame "App.Stop" {
      }
    }
    n68 = case shown="No Error" w62 {
      tunnel: w61 -> [w80 w89]
      tunnel: w60 -> [w79 w87]
      tunnel: [w78 w88] -> w59
      tunnel: [w77 w86] -> w58
      tunnel: w57 -> [w76 _]
      frame No Error {
        n69 = for {
          shift-right: [w83] -> w78
          shift-left: w80 -> [w85]
          shift-right: [w82] -> w77
          shift-left: w79 -> [w84]
          tunnel: w76 -> [w81] mode=indexing
          n70 = Enqueue Element(queue=w85, element=w81, error in (no error)=w84) -> (queue out=w83:refnum<queue>, error out=w82:errorcluster)  [unwired: 1 in, 1 out]
        }
      }
      frame Error {
        n71 = Enqueue Element At Opposite End(queue=w89, element=rqcAlice_States."App.HandleError" ("rqcAlice States"), error in (no error)=w87) -> (queue out=w88:refnum<queue>, error out=w86:errorcluster)  [unwired: 1 in, 1 out]
      }
    }
    n72 = Unbundle By Name(w54) -> ("connected?"=→"connected?":bool)
  }
  n73 = xnode "Close FPGA VI Reference"("FPGA VI Reference In"=w16, "error in"=w15) -> ("error out"=w8:errorcluster)
  n74 = call <vilib>:"Simple Error Handler.vi"("error in (no error)"=w8) -> ()  [unwired: 4 in, 5 out]
